vi "Read Control Metadata.vi"(8 "error in":errorcluster, 10 "control metadata in":T1={"Limit Low"=variant(dbl 0.0), "Limit High"=variant(dbl 0.0), "Min Step"=variant(dbl 0.0)}, 11 "PV Data in":refnum<class "PV Data.lvclass">) -> (0 "error out":errorcluster, 1 "has control metadata?":bool, 2 "control metadata out":T1={"Limit Low"=variant(dbl 0.0), "Limit High"=variant(dbl 0.0), "Min Step"=variant(dbl 0.0)}, 3 "PV Data out":refnum<class "PV Data.lvclass">)   [LabVIEW 2020, in "PV Access.lvlib" / "PV Data.lvlib" / "PV Data.lvclass"]
uses:
  PV Data.lvclass
  Read Field (Variant).vi
  Control Metadata.ctl
  PV Data.lvlib
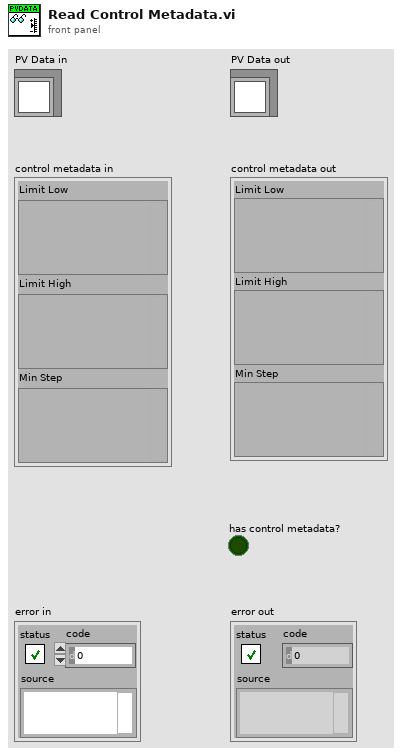
[diagram p1: front panel]
types:
  T1 = typedef "PV Access.lvlib/PV Data.lvlib/Control Metadata.ctl" = cluster{"Limit Low":variant, "Limit High":variant, "Min Step":variant}
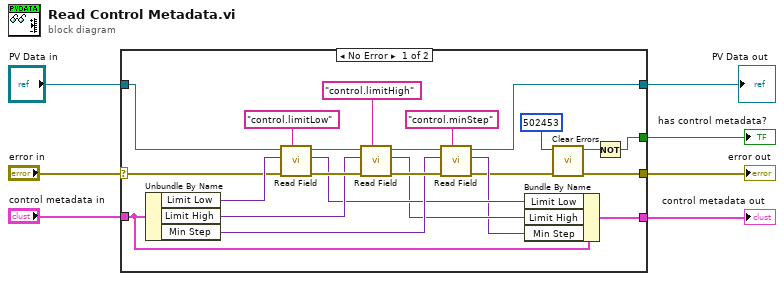
[diagram p0: block diagram]
diagram:
  n1 = case shown="No Error" "error in" {
    selector: "error in" -> [w20 w33]
    tunnel: [w10 w33] -> w7
    tunnel: "PV Data in" -> [w19 w32]
    tunnel: [w12 w32] -> w4
    tunnel: "control metadata in" -> [w18 w31]
    tunnel: [w14 w31] -> w2
    tunnel: [w8 _] -> w1
    frame No Error {
      n2 = Unbundle By Name(w18) -> ("Limit Low"=w23:variant, "Limit High"=w21:variant, "Min Step"=w22:variant)
      n3 = call-poly "Read Field.vi"("field name"="control.limitLow", "error in (no error)"=w20, "value"=w23, "PV Data in"=w19) -> ("error out"=w30:errorcluster, "value out"=w17:variant, "PV Data out"=w27:refnum<class "PV Data.lvclass">)  [unwired: 4 in, 1 out]
      n4 = call-poly "Read Field.vi"("field name"="control.limitHigh", "error in (no error)"=w30, "value"=w21, "PV Data in"=w27) -> ("error out"=w29:errorcluster, "value out"=w16:variant, "PV Data out"=w28:refnum<class "PV Data.lvclass">)  [unwired: 4 in, 1 out]
      n5 = call-poly "Read Field.vi"("field name"="control.minStep", "error in (no error)"=w29, "value"=w22, "PV Data in"=w28) -> ("error out"=w11:errorcluster, "value out"=w15:variant, "PV Data out"=w12:refnum<class "PV Data.lvclass">)  [unwired: 4 in, 1 out]
      n6 = Bundle By Name(cluster=w18, "Limit Low"=w17, "Limit High"=w16, "Min Step"=w15) -> (w14:T1)
      n7 = call <vilib>:"Clear Errors.vi"("error in (no error)"=w11, "specific error code to clear (0: all)"=502453) -> ("error out"=w10:errorcluster, "specific error cleared?"=w9:bool)  [unwired: 4 in]
      n8 = Not(x=w9) -> (.not. x?=w8:bool)
    }
    frame Error {
    }
  }
  "error out" <- w7
  "PV Data out" <- w4
  "has control metadata?" <- w1
  "control metadata out" <- w2
